vi "handleRuntimeMenuSelection.vi"(8 "error in (no error)":errorcluster, 10 "ItemPath":string, 11 "QControl_Graph in":refnum<class "QControl_Graph.lvclass">) -> (0 "error out":errorcluster, 3 "QControl_Graph out":refnum<class "QControl_Graph.lvclass">)   [LabVIEW 2017, in "QControl_Graph.lvclass"]
uses:
  QControl_Graph.lvclass
  Actions.ctl
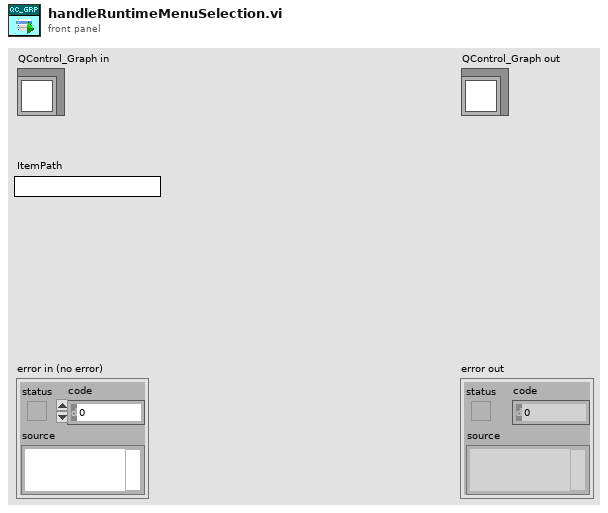
[diagram p1: front panel]
types:
  T1 = typedef "QControl_Graph.lvclass/Actions.ctl" = enum16{"Undefined", "BGK Color", "Highlight Plot", "Mouse Zoom", "Show Cursors", "Cursor Properties", "Show Markers"}
  T2 = typedef "QControl_Graph.lvclass/Cursor Properties.ctl" = cluster{"Horizontal Line?":bool, "Vertical Line?":bool, "Timestamp":enum16{"at TOP", "at BOTTOM", "none"}, "time format (%H:%M:%S)":string, "size":i16, "font":T3, "alignment(left, top)":T4, "TextFormat":string}
  T3 = typedef "QControl_Graph.lvclass/Font.ctl" = cluster{"Font Name":string, "Size":i16, "Strikeout?":bool, "Italic?":bool, "Underline?":bool, "Outline?":bool, "Shadow":bool, "Bold?":bool}
  T4 = typedef "QControl_Graph.lvclass/Alignment.ctl" = cluster{"Horizontal":T5, "Vertical":T6}
  T5 = typedef "QControl_Graph.lvclass/Alignment.Horizontal.ctl" = enum16{"left", "center", "right"}
  T6 = typedef "QControl_Graph.lvclass/Alignment.Vertical.ctl" = enum16{"top", "center", "bottom"}
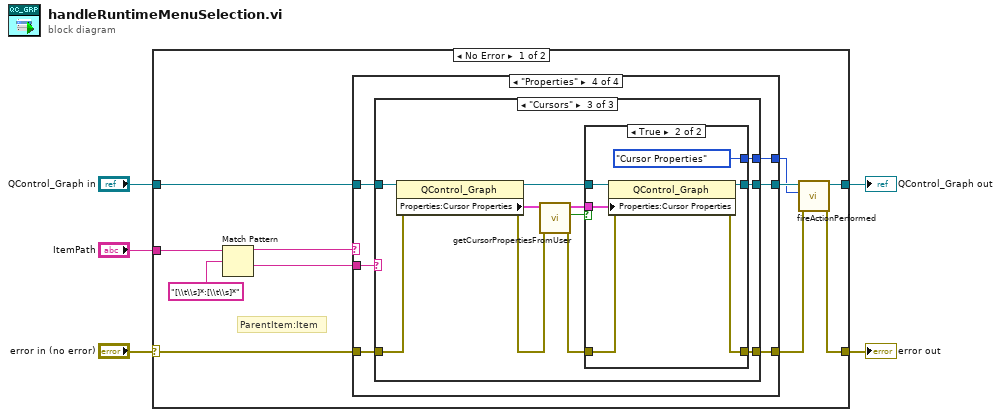
[diagram p0: block diagram]
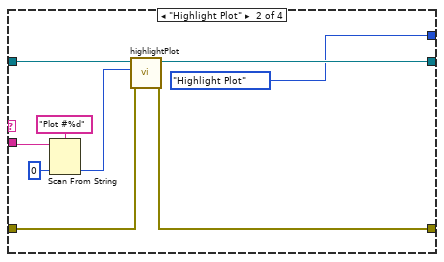
[diagram p3: hidden frame]
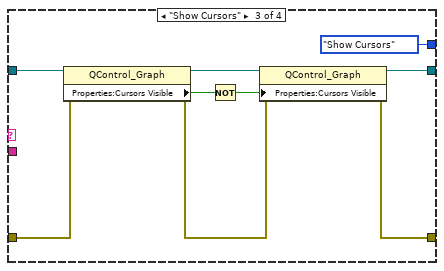
[diagram p4: hidden frame]
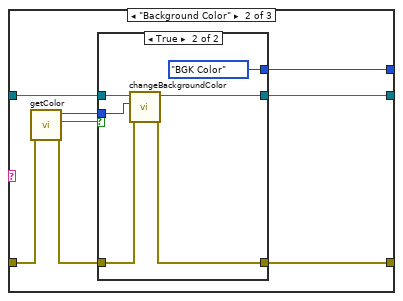
[diagram p6: hidden frame]
diagram:
  n1 = case shown="No Error" "error in (no error)" {
    selector: "error in (no error)" -> [w11 w81]
    tunnel: [w6 w81] -> w4
    tunnel: [w9 w80] -> w2
    tunnel: "QControl_Graph in" -> [w12 w80]
    tunnel: "ItemPath" -> [w15 _]
    frame No Error {
      # "ParentItem:Item"
      n2 = Match Pattern(string=w15, regular expression="[\\t\\s]*:[\\t\\s]*") -> (before substring=w14:string, after substring=w13:string)  [unwired: 1 in, 2 out]
      n3 = case shown="\"Properties\"" w14 {
        tunnel: w13 -> [_ w27 _ w37]
        tunnel: w12 -> [w18 w23 w32 w42]
        tunnel: [w18 w22 w35 w41] -> w10
        tunnel: w11 -> [w17 w21 w29 w38]
        tunnel: [w17 w20 w34 w40] -> w7
        tunnel: [_ Actions."Highlight Plot" ("Actions") Actions."Show Cursors" ("Actions") w39] -> w8
        frame Default {
        }
        frame "Highlight Plot" {
          n4 = Scan From String(format string="Plot #%d", input string=w27, default 1=u32 0 ("default value 1")) -> (output 1=w24:u32)  [unwired: 2 in, 3 out]
          n5 = call-dynamic "highlightPlot.vi"("error in (no error)"=w21, "PlotNum"=w24, "QControl_Graph in"=w23) -> ("error out"=w20:errorcluster, "QControl_Graph out"=w22:refnum<class "QControl_Graph.lvclass">)  [unwired: 7 in]
        }
        frame "Show Cursors" {
          n6 = property class="QControl_Graph"(reference=w32, error in=w29) -> (reference out=w33:refnum<class "QControl_Graph.lvclass">, error out=w28:errorcluster, "Properties:Cursors Visible"=w31:bool)
          n7 = Not(x=w31) -> (.not. x?=w30:bool)
          n8 = property class="QControl_Graph"(reference=w33, error in=w28, "Properties:Cursors Visible"=w30) -> (reference out=w35:refnum<class "QControl_Graph.lvclass">, error out=w34:errorcluster)
        }
        frame "Properties" {
          n9 = case shown="\"Cursors\"" w37 {
            tunnel: w42 -> [w44 w52 w71]
            tunnel: [w44 w51 w67] -> w41
            tunnel: [w43 w50 w66] -> w40
            tunnel: [_ w49 w62] -> w39
            tunnel: w38 -> [w43 w48 w63]
            frame Default {
            }
            frame "Background Color" {
              n10 = call "getColor.vi"("error in (no error)"=w48) -> ("error out"=w47:errorcluster, "ok"=w45:bool, "Color"=w46:u32)  [unwired: 8 in]
              n11 = case shown="True" w45 {
                tunnel: w52 -> [w54 w60]
                tunnel: [w54 w59] -> w51
                tunnel: [w53 w58] -> w50
                tunnel: [_ Actions."BGK Color" ("Actions")] -> w49
                tunnel: w47 -> [w53 w56]
                tunnel: w46 -> [_ w55]
                frame False {
                  # "Cancelled or\nwindow closed"
                }
                frame True {
                  n12 = call-dynamic "changeBackgroundColor.vi"("error in (no error)"=w56, "Color (transparent)"=w55, "QControl_Graph in"=w60) -> ("error out"=w58:errorcluster, "QControl_Graph out"=w59:refnum<class "QControl_Graph.lvclass">)  [unwired: 7 in]
                }
              }
            }
            frame "Cursors" {
              n13 = property class="QControl_Graph"(reference=w71, error in=w63) -> (reference out=w70:refnum<class "QControl_Graph.lvclass">, error out=w64:errorcluster, "Properties:Cursor Properties"=w69:T2)
              n14 = call "getCursorPropertiesFromUser.vi"("error in (no error)"=w64, "Cursor Properties in"=w69) -> ("error out"=w65:errorcluster, "ok"=w61:bool, "Cursor Properties out"=w68:T2)  [unwired: 7 in]
              n15 = case shown="True" w61 {
                tunnel: w70 -> [w73 w79]
                tunnel: w68 -> [_ w78]
                tunnel: [w73 w77] -> w67
                tunnel: [w72 w76] -> w66
                tunnel: w65 -> [w72 w75]
                tunnel: [_ Actions."Cursor Properties" ("Actions")] -> w62
                frame False {
                }
                frame True {
                  n16 = property class="QControl_Graph"(reference=w79, error in=w75, "Properties:Cursor Properties"=w78) -> (reference out=w77:refnum<class "QControl_Graph.lvclass">, error out=w76:errorcluster)
                }
              }
            }
          }
        }
      }
      n17 = call-dynamic "fireActionPerformed.vi"("error in (no error)"=w7, "Action"=w8, "QControl_Graph in"=w10) -> ("error out"=w6:errorcluster, "QControl_Graph out"=w9:refnum<class "QControl_Graph.lvclass">)  [unwired: 7 in]
    }
    frame Error {
    }
  }
  "error out" <- w4
  "QControl_Graph out" <- w2
